vi "Test Set Pin Status Command.vi"(8 "error in (no error)":errorcluster, 11 "TestCase in":refnum<class "Test Set Pin Status Command.lvclass">) -> (0 "error out":errorcluster, 3 "TestCase out":refnum<class "Test Set Pin Status Command.lvclass">)   [LabVIEW 2020, in "Test Set Pin Status Command.lvclass"]
uses:
  Test Set Pin Status Command.lvclass
  Implementations/Simulado/Simulado.lvclass
  <vilib>/addons/_JKI Toolkits/VI Tester/TestCase.llb/TestCase.lvclass
  C:/Program Files (x86)/National Instruments/LabVIEW 2020/vi.lib/addons/_JKI Toolkits/VI Tester/TestCase.llb/TestCase.lvclass
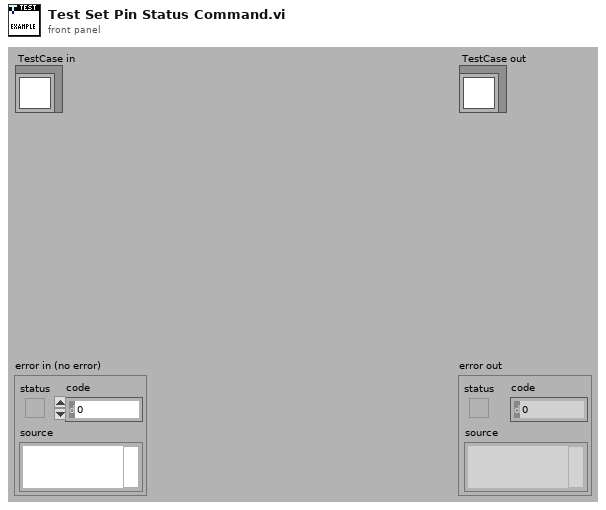
[diagram p1: front panel]
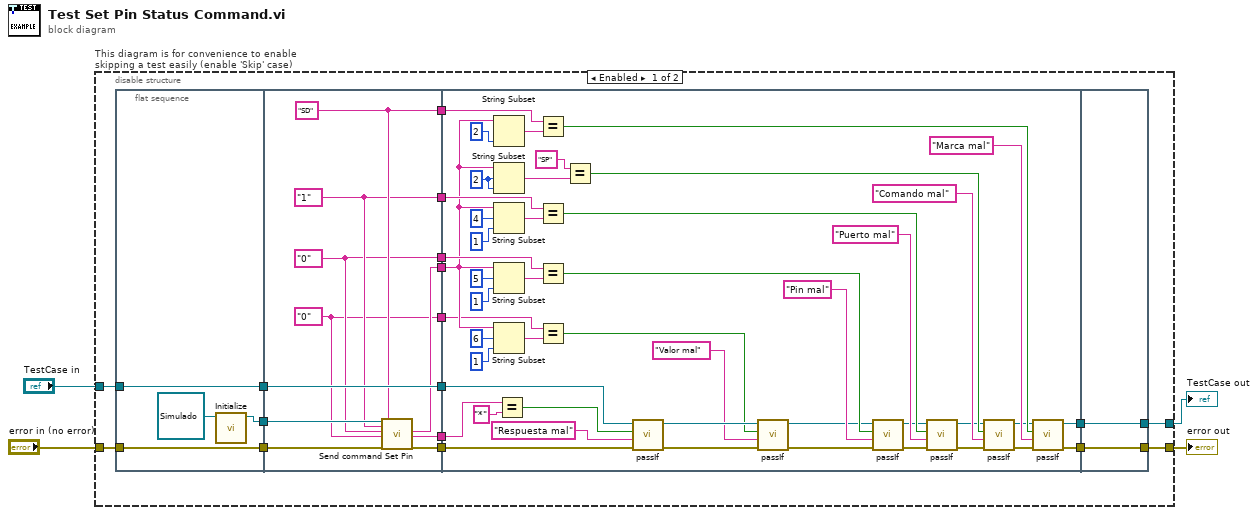
[diagram p0: block diagram]
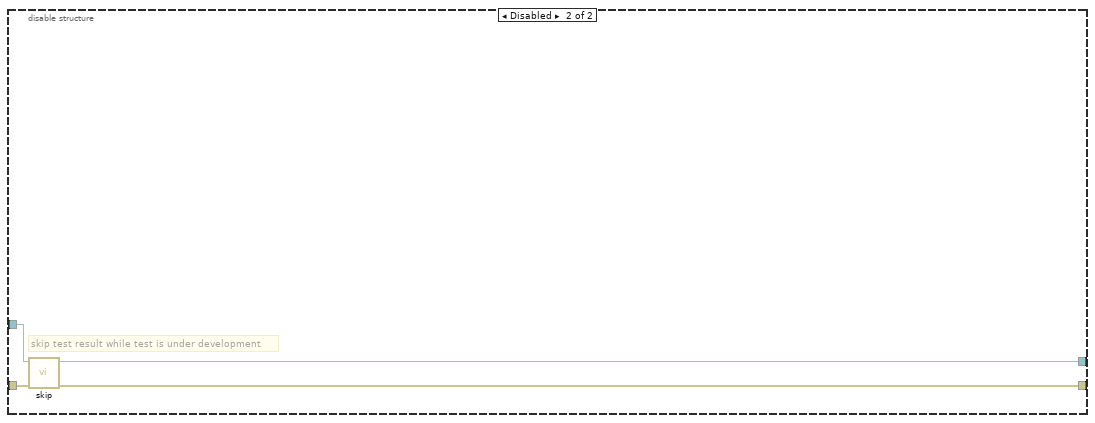
[diagram p2: hidden frame]
diagram:
  n1 = disable-structure "This diagram is for convenience to enable skipping a test easily (enable 'Skip' case)" shown="Enabled" {
    disable-tunnel: "TestCase in" -> [w11 w88]
    disable-tunnel: [w8 w86] -> w1
    disable-tunnel: [w9 w87] -> w3
    disable-tunnel: "error in (no error)" -> [w10 w85]
    frame Enabled {
      n2 = flat-sequence {
        tunnel: w11 -> [w25]
        tunnel: [w25] -> w21
        tunnel: w10 -> [w24]
        tunnel: [w24] -> w20
        tunnel: [w22] -> w19
        tunnel: [w35] -> w18
        tunnel: w21 -> [w35]
        tunnel: [w32] -> w17
        tunnel: w20 -> [w31]
        tunnel: w19 -> [w30]
        tunnel: [w34] -> w16
        tunnel: [w33] -> w15
        tunnel: [w29] -> w14
        tunnel: [w28] -> w7
        tunnel: [w27] -> w6
        tunnel: [w26] -> w5
        tunnel: [w79] -> w13
        tunnel: w18 -> [w66]
        tunnel: [w78] -> w12
        tunnel: w17 -> [w65]
        tunnel: w16 -> [w43]
        tunnel: w15 -> [w68]
        tunnel: w14 -> [w80]
        tunnel: w7 -> [w57]
        tunnel: w6 -> [w51]
        tunnel: w5 -> [w42]
        tunnel: [w84] -> w8
        tunnel: w13 -> [w84]
        tunnel: [w83] -> w9
        tunnel: w12 -> [w83]
        frame #0 {
          n3 = call-dynamic "Initialize.vi"("object in"=refnum<class "Simulado.lvclass"> refnum ("Simulado.lvclass")) -> ("object out"=w22:refnum<class "Simulado.lvclass">)  [unwired: 9 in, 1 out]
        }
        frame #1 {
          w26 = "0" ("Valor")
          w27 = "0" ("Pin")
          w28 = "1" ("Puerto")
          w29 = "SD" ("Marca")
          n4 = call-dynamic "Send command Set Pin.vi"("Simulado in"=w30, "Puerto"=w28, "Pin"=w27, "Valor"=w26, "error in (no error)"=w31, "Marca"=w29) -> ("Command"=w34:string, "Expected response"=w33:string, "error out"=w32:errorcluster)  [unwired: 10 in, 1 out]
        }
        frame #2 {
          w75 = 2 ("length (rest)")
          n5 = String Subset(string=w43, length (rest)=2 ("length (rest)")) -> (substring=w81:string)  [unwired: 1 in]
          n6 = String Subset(string=w43, offset (0)=w75, length (rest)=w75) -> (substring=w74:string)
          n7 = String Subset(string=w43, offset (0)=4, length (rest)=1 ("length (rest)")) -> (substring=w62:string)
          n8 = String Subset(string=w43, offset (0)=5, length (rest)=1 ("length (rest)")) -> (substring=w54:string)
          n9 = String Subset(string=w43, offset (0)=6, length (rest)=1 ("length (rest)")) -> (substring=w46:string)
          n10 = Equal?(x=w68, y="*") -> (x = y?=w64:bool)
          n11 = Equal?(x=w80, y=w81) -> (x = y?=w77:bool)
          n12 = Equal?(x=w57, y=w62) -> (x = y?=w56:bool)
          n13 = Equal?(x=w51, y=w54) -> (x = y?=w48:bool)
          n14 = Equal?(x=w42, y=w46) -> (x = y?=w37:bool)
          n15 = Equal?(x="SP", y=w74) -> (x = y?=w70:bool)
          n16 = call-dynamic "passIf.vi"("error in (no error)"=w65, "message (\"\")"="Respuesta mal" ("message (\"\")"), "pass"=w64, "TestCase in"=w66) -> ("error out"=w38:errorcluster, "TestCase out"=w39:refnum<class "Test Set Pin Status Command.lvclass">)  [unwired: 6 in]
          n17 = call-dynamic "passIf.vi"("error in (no error)"=w38, "message (\"\")"="Valor mal" ("message (\"\")"), "pass"=w37, "TestCase in"=w39) -> ("error out"=w41:errorcluster, "TestCase out"=w40:refnum<class "Test Set Pin Status Command.lvclass">)  [unwired: 6 in]
          n18 = call-dynamic "passIf.vi"("error in (no error)"=w41, "message (\"\")"="Pin mal" ("message (\"\")"), "pass"=w48, "TestCase in"=w40) -> ("error out"=w50:errorcluster, "TestCase out"=w49:refnum<class "Test Set Pin Status Command.lvclass">)  [unwired: 6 in]
          n19 = call-dynamic "passIf.vi"("error in (no error)"=w50, "message (\"\")"="Puerto mal" ("message (\"\")"), "pass"=w56, "TestCase in"=w49) -> ("error out"=w60:errorcluster, "TestCase out"=w59:refnum<class "Test Set Pin Status Command.lvclass">)  [unwired: 6 in]
          n20 = call-dynamic "passIf.vi"("error in (no error)"=w60, "message (\"\")"="Comando mal" ("message (\"\")"), "pass"=w70, "TestCase in"=w59) -> ("error out"=w71:errorcluster, "TestCase out"=w72:refnum<class "Test Set Pin Status Command.lvclass">)  [unwired: 6 in]
          n21 = call-dynamic "passIf.vi"("error in (no error)"=w71, "message (\"\")"="Marca mal" ("message (\"\")"), "pass"=w77, "TestCase in"=w72) -> ("error out"=w78:errorcluster, "TestCase out"=w79:refnum<class "Test Set Pin Status Command.lvclass">)  [unwired: 6 in]
        }
        frame #3 {
        }
      }
    }
    frame Disabled {
      # "skip test result while test is under development"
      n22 = call <vilib>:"skip.vi"("error in (no error)"=w85, "TestCase in"=w88) -> ("error out"=w87:errorcluster, "TestCase out"=w86:refnum<class "Test Set Pin Status Command.lvclass">)  [unwired: 8 in]
    }
  }
  "error out" <- w3
  "TestCase out" <- w1
